vi "NATS UNSUB.vi"(6 "timeout ms (conn default)":i32=-2, 8 "error in":errorcluster, 9 "After n messages (0: Immediate)":u32, 10 "sub id":string, 11 "nats connection in":T1={"connection ID"=refnum, "server INFO"="", "timeout ms"=5000, "verbose?"=FALSE, "server headers?"=FALSE, "client headers?"=FALSE}) -> (0 "error out":errorcluster, 3 "dup nats connection":T1={"connection ID"=refnum, "server INFO"="", "timeout ms"=5000, "verbose?"=FALSE, "server headers?"=FALSE, "client headers?"=FALSE})   [LabVIEW 2013, in "NATS Core.lvlib"]
doc: "Unsubscribes from the specified subscription ID."
uses:
  NATS Core.lvlib
  Controls/nats connection.ctl
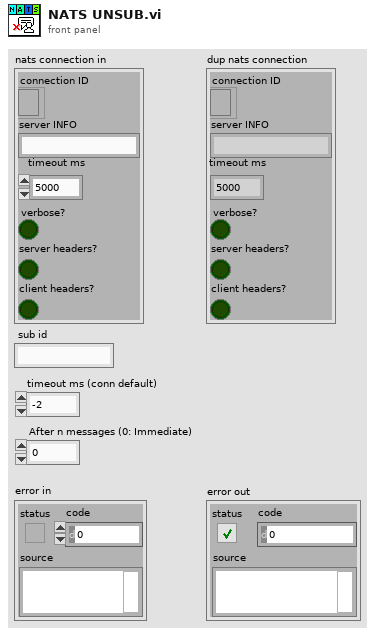
[diagram p1: front panel]
types:
  T1 = typedef "NATS Core.lvlib/nats connection.ctl" = cluster{"connection ID":refnum<k5>, "server INFO":string, "timeout ms":i32, "verbose?":bool, "server headers?":bool, "client headers?":bool}
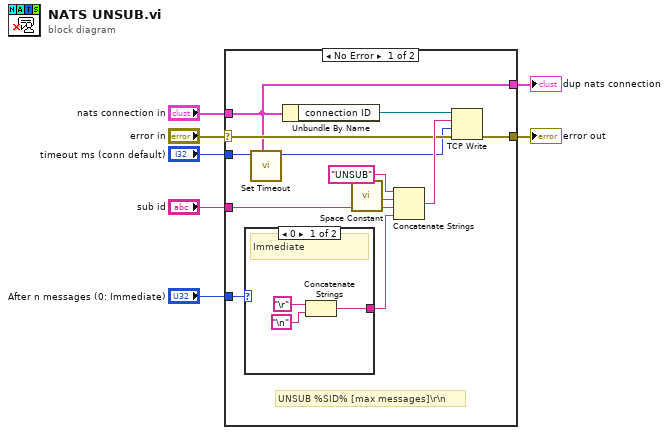
[diagram p0: block diagram]
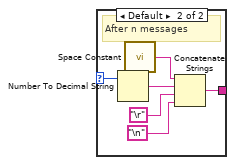
[diagram p2: hidden frame]
diagram:
  n1 = case shown="No Error" "error in" {
    selector: "error in" -> [w13 w30]
    tunnel: "timeout ms (conn default)" -> [w9 _]
    tunnel: [w18 w30] -> w6
    tunnel: "sub id" -> [w17 _]
    tunnel: "nats connection in" -> [w10 w29]
    tunnel: "After n messages (0: Immediate)" -> [w12 _]
    tunnel: [w10 w29] -> w1
    frame No Error {
      # "UNSUB %SID% [max messages]\\r\\n"
      n2 = case shown="0" w12 {
        selector: w12 -> [_ w25]
        tunnel: [w20 w26] -> w11
        frame 0 {
          # "Immediate"
          n3 = Concatenate Strings("\r", "\n") -> (w20:string)
        }
        frame Default {
          # "After n messages"
          n4 = Number To Decimal String(number=w25) -> (decimal integer string=w24:string)  [unwired: 1 in]
          n5 = call <vilib>:"Space Constant.vi"() -> ("String"=w23:string)
          n6 = Concatenate Strings(w23, w24, "\r", "\n") -> (w26:string)
        }
      }
      n7 = call "Set Timeout.vi"("nats connection in"=w10, "timeout ms in"=w9) -> ("timeout ms out"=w8:i32)  [unwired: 9 in]
      n8 = Unbundle By Name(w10) -> ("connection ID"=w19:refnum<k5>)
      n9 = call <vilib>:"Space Constant.vi"() -> ("String"=w15:string)
      n10 = Concatenate Strings("UNSUB", w15, w17, w11) -> (w14:string)
      n11 = TCP Write(connection ID=w19, data in=w14, error in (no error)=w13, 9:w8) -> (error out=w18:errorcluster)  [unwired: 2 out]
    }
    frame Error {
    }
  }
  "dup nats connection" <- w1
  "error out" <- w6
